vi "FindArduino.vi"() -> (2 "VISA resource name":refnum<visa-resource-name>)   [LabVIEW 2014]
panel:
  out "Array":string[](array[string])
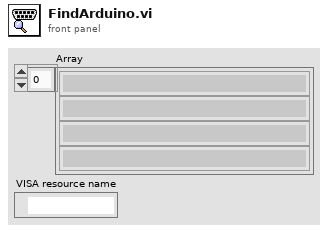
[diagram p1: front panel]
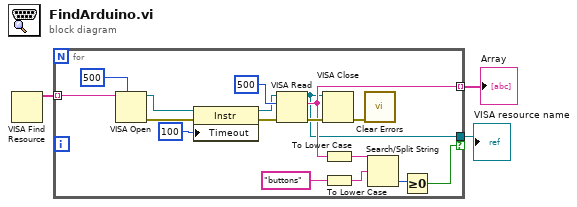
[diagram p0: block diagram]
diagram:
  n1 = VISA Find Resource() -> (3:w3:string[])  [unwired: 3 in, 2 out]
  n2 = for {
    tunnel: w3 -> [w20] mode=indexing
    tunnel: [w10] -> w2 mode=indexing
    tunnel: [w8] -> w1 if=w4
    n3 = VISA Open(timeout (0)=u32 500 ("VISA Open timeout (0)"), VISA resource name=w20) -> (VISA resource name=w19:refnum<visa-resource-name>, error out=w12:errorcluster)  [unwired: 3 in]
    n4 = property class="Instr"(reference=w19, error in=w12, "Timeout"=u32 100 ("General Settings:Timeout Value")) -> (reference out=w14:refnum<visa-resource-name>, error out=w11:errorcluster)
    n5 = VISA Read(VISA resource name=w14, byte count=u32 500, error in (no error)=w11) -> (VISA resource name out=w8:refnum<visa-resource-name>, read buffer=w10:string, error out=w17:errorcluster)  [unwired: 1 out]
    n6 = VISA Close(VISA resource name=w8, error in (no error)=w17) -> (error out=w16:errorcluster)
    n7 = To Lower Case(string=w10) -> (all lower case string=w7:string)
    n8 = To Lower Case(string="buttons") -> (all lower case string=w6:string)
    n9 = call <vilib>:"Clear Errors.vi"("error in (no error)"=w16) -> ()  [unwired: 5 in, 2 out]
    n10 = Search/Split String(string=w7, search string/char (-)=w6) -> (offset of match=w5:i32)  [unwired: 1 in, 2 out]
    n11 = Greater Or Equal To 0?(x=w5) -> (x >= 0?=w4:bool)
  }
  "Array" <- w2
  "VISA resource name" <- w1
